vi "Read INI File.vi"(8 "error in":errorcluster, 11 "Path":path) -> (0 "error out":errorcluster, 1 "Modbus Configuration":T1, 2 "DER_Info":T3)   [LabVIEW 2018, in "AE75TX Actor.lvlib" / "AE75TX.lvclass"]
uses:
  AE75TX.lvclass
  <vilib>/ORNL/CSEISMIC DDS/CSEISMIC DDS Base/Data Types/DER_Info.ctl
  <vilib>/ORNL/CSEISMIC DDS/CSEISMIC DDS Base/Data Types/Controls/DeviceID.ctl
  Controls/Modbus Configuration Cluster.ctl
  <vilib>/Utility/config.llb/NI_LVConfig.lvlib
  <vilib>/ORNL/CSEISMIC DDS/CSEISMIC DDS Base/CSEISMIC DDS.lvclass
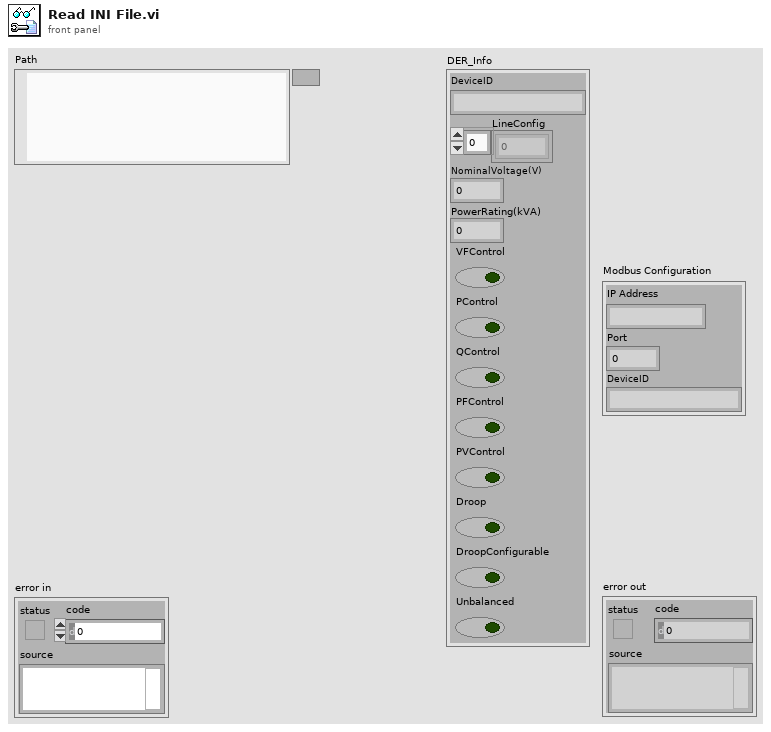
[diagram p1: front panel]
types:
  T1 = typedef "AE75TX Actor.lvlib/AE75TX.lvclass/Modbus Configuration Cluster.ctl" = cluster{"IP Address":string, "Port":u16, "DeviceID":T2}
  T2 = typedef "CSEISMIC DDS.lvlib/CSEISMIC DDS.lvclass/DeviceID.ctl" = string
  T3 = typedef "CSEISMIC DDS.lvlib/CSEISMIC DDS.lvclass/DER_Info.ctl" = cluster{"DeviceID":T2, "LineConfig":u8[], "NominalVoltage(V)":dbl, "PowerRating(kVA)":dbl, "VFControl":bool, "PControl":bool, "QControl":bool, "PFControl":bool, "PVControl":bool, "Droop":bool, "DroopConfigurable":bool, "Unbalanced":bool}
  T4 = typedef "NI_LVConfig.lvlib/Config Data RefNum.ctl" = refnum<k1>
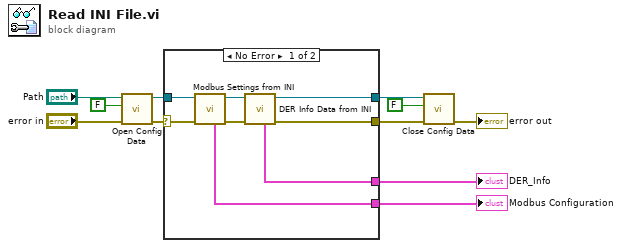
[diagram p0: block diagram]
diagram:
  n1 = call <vilib>:"Open Config Data.vi"("error in (no error)"="error in", "create file if necessary (T)"=FALSE, "configuration file path"="Path") -> ("error out"=w9:errorcluster, "refnum"=w8:T4)  [unwired: 6 in, 1 out]
  n2 = case shown="No Error" w9 {
    selector: w9 -> [w15 w20]
    tunnel: w8 -> [w16 w21]
    tunnel: [w19 w21] -> w7
    tunnel: [w18 w20] -> w6
    tunnel: [w17 _] -> w2
    tunnel: [w12 _] -> w1
    frame No Error {
      n3 = call "Modbus Settings from INI.vi"("error in"=w15, "Config Refnum in"=w16) -> ("error out"=w14:errorcluster, "Config Refnum out"=w13:T4, "Modbus Configuration"=w12:T1)  [unwired: 7 in]
      n4 = call "DER Info Data from INI.vi"("error in"=w14, "Config Refnum in"=w13) -> ("error out"=w18:errorcluster, "Config Refnum out"=w19:T4, "DER_Info"=w17:T3)  [unwired: 7 in]
    }
    frame Error {
    }
  }
  "DER_Info" <- w2
  "Modbus Configuration" <- w1
  n5 = call <vilib>:"Close Config Data.vi"("error in (no error)"=w6, "write file if changed (T)"=FALSE, "refnum"=w7) -> ("error out"=→"error out":errorcluster)  [unwired: 7 in, 1 out]
